vi "DATA_ANALYSIS.vi"() -> ()   [LabVIEW 2019]
uses:
  <vilib>/numeric/Random Number (Range) DBL.vi
panel:
  out "Waveform Graph":dbl[][](graph)
  in  "stop":bool
  out "OUTPUT":string
  out "A>B":bool
  out "CITY B":dbl
  out "Thermometer 2":dbl(slide) scale=0.0..100.0
  out "Thermometer":dbl(slide) scale=0.0..100.0
  out "CITY A":dbl
  # "TEMPERATURE MONITORING"
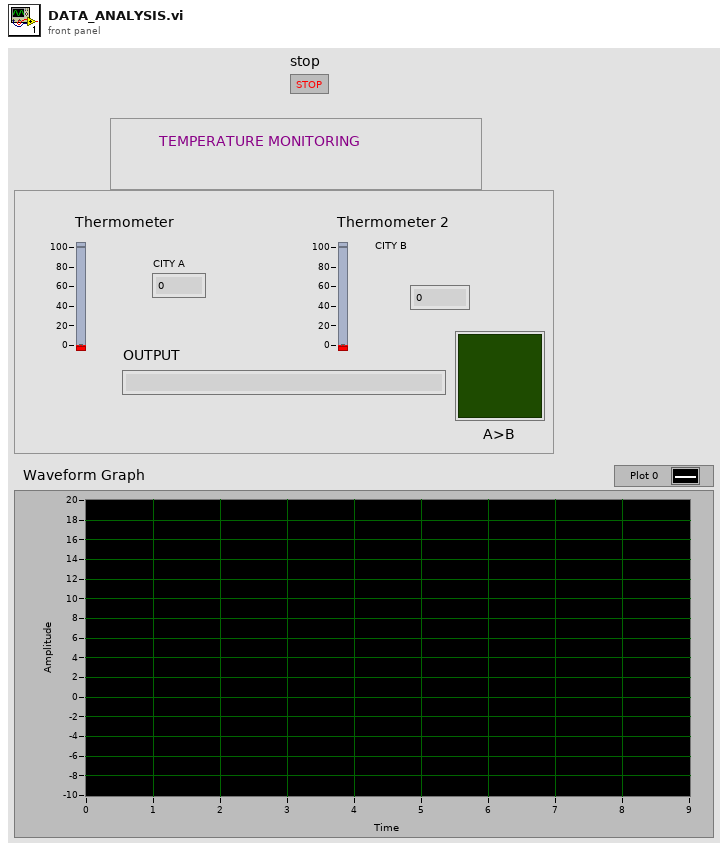
[diagram p1: front panel]
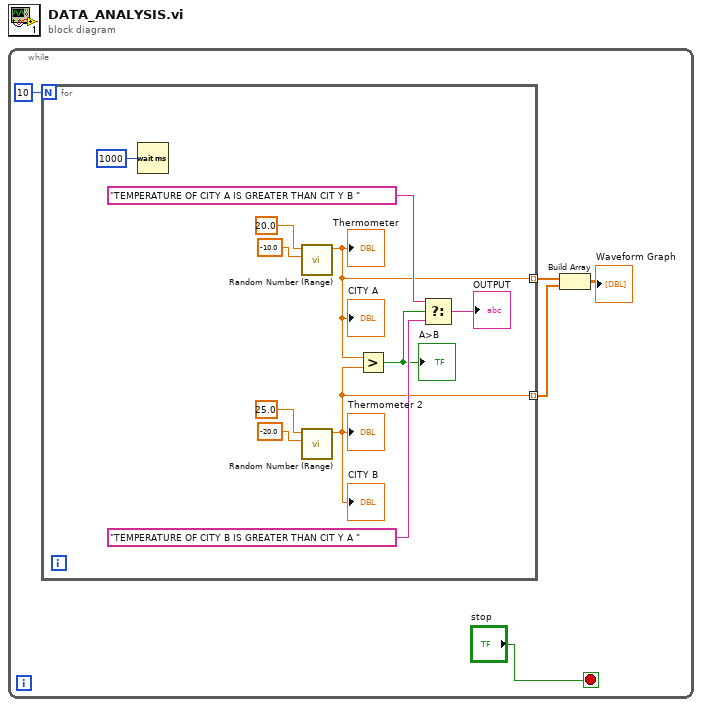
[diagram p0: block diagram]
diagram:
  n1 = while {
    stop <- "stop" stop-if-true
    n2 = for {
      N: 10 -> [_]
      tunnel: [w7] -> w4 mode=indexing
      tunnel: [w6] -> w3 mode=indexing
      n3 = Wait (ms)(milliseconds to wait=u32 1000 ("millisecond timer value")) -> ()  [unwired: 1 out]
      n4 = call-poly <vilib>:"Random Number (Range).vi"("lower bound (0)"=-10.0, "upper bound (100)"=20.0) -> ("number"=w7:dbl)  [unwired: 9 in]
      "CITY A" <- w7
      "Thermometer" <- w7
      n5 = call-poly <vilib>:"Random Number (Range).vi"("lower bound (0)"=-20.0, "upper bound (100)"=25.0) -> ("number"=w6:dbl)  [unwired: 9 in]
      "CITY B" <- w6
      "Thermometer 2" <- w6
      n6 = Greater?(x=w7, y=w6) -> (0:w8:bool)
      "A>B" <- w8
      n7 = Select(t="TEMPERATURE OF CITY A IS GREATER THAN CIT Y B ", s=w8, f="TEMPERATURE OF CITY B IS GREATER THAN CIT Y A ") -> (s? t:f=→"OUTPUT":string)
    }
    n8 = Build Array(w4, w3) -> (→"Waveform Graph":dbl[][])
  }
